vi "HEWH LowerHeater On.vi"(0 "VISA session":refnum<visa-resource-name>="MW100", 2 "Semiphore":T1, 5 "Output Data":string[][](array[string]), 7 "StdElecric?":bool, 11 "Error In":errorcluster) -> (4 "dup VISA session":refnum<visa-resource-name>, 6 "Value":bool, 15 "error out":errorcluster)   [LabVIEW 2009]
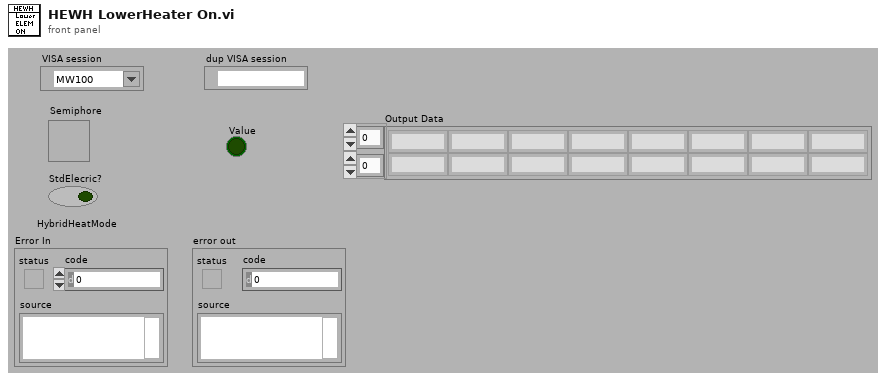
[diagram p1: front panel]
types:
  T1 = typedef "Semaphore RefNum" = refnum<k1>
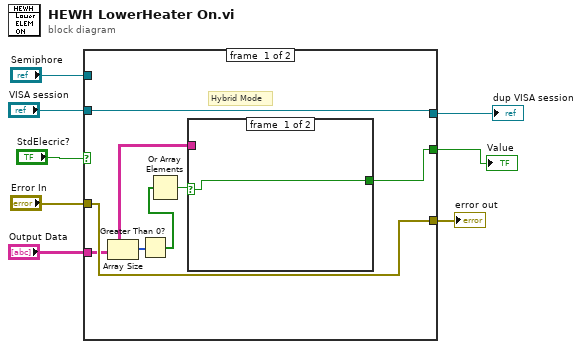
[diagram p0: block diagram]
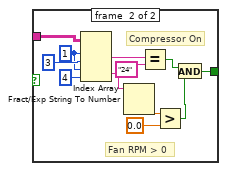
[diagram p2: hidden frame]
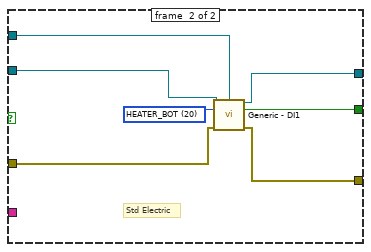
[diagram p3: hidden frame]
diagram:
  n1 = case shown="False" "StdElecric?" {
    tunnel: "VISA session" -> [w15 w34]
    tunnel: "Semiphore" -> [_ w33]
    tunnel: "Error In" -> [w13 w32]
    tunnel: [w13 w31] -> w4
    tunnel: [w15 w30] -> w3
    tunnel: [w14 w29] -> w2
    tunnel: "Output Data" -> [w12 _]
    frame #0 {
      # "Hybrid Mode"
      n2 = Array Size(array=w12) -> (size(s)=w11:i32[])
      n3 = Greater Than 0?(x=w11) -> (x > 0?=w10:bool[])
      n4 = Or Array Elements(Boolean array=w10) -> (logical OR=w9:bool)
      n5 = case shown="False" w9 {
        selector: w9 -> [w16 _]
        tunnel: [w16 w18] -> w14
        tunnel: w12 -> [_ w17]
        frame #0 {
        }
        frame #1 {
          w24 = 1 ("index (row)")
          # "Compressor On"
          # "Fan RPM > 0"
          n6 = Index Array(array=w17, index (row) #1=w24, index (col) #1=3 ("disabled index (col)"), index (row) #2=w24, index (col) #2=4 ("disabled index (col)")) -> (element #1=w27:string, element #2=w22:string)
          n7 = Fract/Exp String To Number(string=w22) -> (number=w21:dbl)  [unwired: 3 in, 1 out]
          n8 = Equal?(x=w27, y="24") -> (x = y?=w25:bool)
          n9 = Greater?(x=w21, y=0.0) -> (0:w19:bool)
          n10 = And(x=w25, y=w19) -> (x .and. y?=w18:bool)
        }
      }
    }
    frame #1 {
      w35 = u16 20 items=["RTD_IN", "RTD_OUT", "RTD_AMB", "Tc_1", "Tc_2", "Tc_3", "Tc_4", "Tc_5", "Tc_6", "Tc_down", "Pres_HI1", "Pres_HI2", "Pres_LOW", "VLV_IN", "VLV_3W", "VLV_OUT", "PWR_MAIN", "FLOWMETER", "4-20_OUT", "HEATER_TOP", "HEATER_BOT", "COMPRESSOR", "DRM_LOW", "DRM_HIGH", "INTF_TEMPFLO", "INTF_READY", "INTF_START", "INTF_STOP"] ("Channel_Enum")
      # "Std Electric"
      n11 = call "Generic - DI1.vi"("VISA session"=w34, "Semiphore"=w33, "Channel_Enum"=w35, "Error In"=w32) -> ("dup VISA session"=w30:refnum<visa-resource-name>, "Value"=w29:bool, "error out"=w31:errorcluster)  [unwired: 9 in]
    }
  }
  "error out" <- w4
  "dup VISA session" <- w3
  "Value" <- w2
